vi "Dwell.vi"(8 "error in":errorcluster, 10 "Parameters":dbl[](array[numeric]), 11 "Events":i32[](array[numeric])) -> (0 "error out":errorcluster)   [LabVIEW 2013]
uses:
  NIST2/Arm Globals.vi
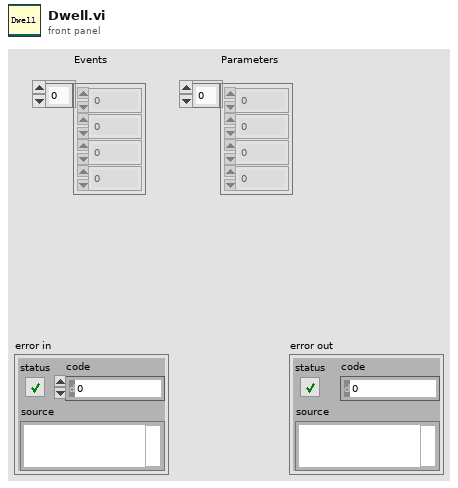
[diagram p1: front panel]
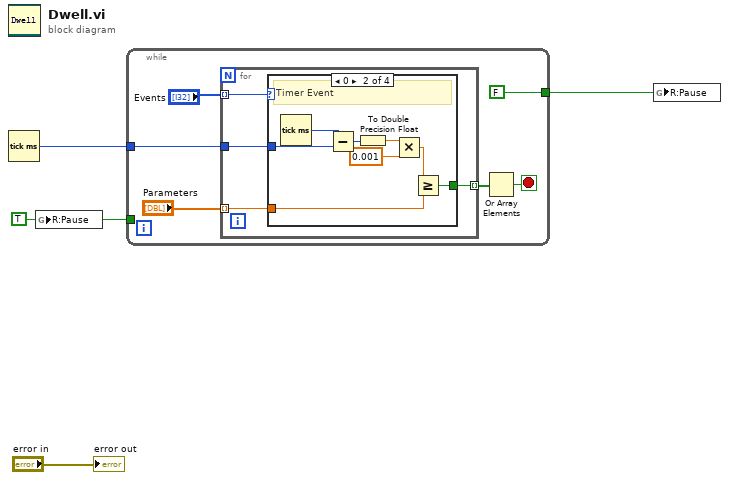
[diagram p0: block diagram]
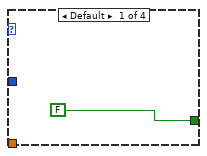
[diagram p2: hidden frame]
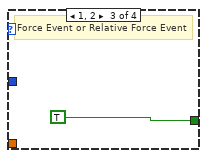
[diagram p3: hidden frame]
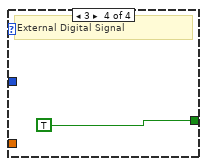
[diagram p4: hidden frame]
diagram:
  w2 = TRUE ("R:Pause")
  n1 = Tick Count (ms)() -> (millisecond timer value=w3:u32)
  n2 = global write "Arm Globals.vi" "R:Pause"(w2) -> ()
  n3 = while {
    tunnel: w3 -> [w8]
    tunnel: w2 -> [_]
    tunnel: [FALSE] -> w1
    stop <- w6 stop-if-true
    n4 = for {
      tunnel: "Events" -> [w14] mode=indexing
      tunnel: "Parameters" -> [w13] mode=indexing
      tunnel: w8 -> [w12]
      tunnel: [w11] -> w7 mode=indexing
      n5 = case shown="0" w14 {
        tunnel: w13 -> [_ w17 _ _]
        tunnel: w12 -> [_ w22 _ _]
        tunnel: [FALSE w16 TRUE TRUE] -> w11
        frame Default {
        }
        frame 0 {
          # "Timer Event"
          n6 = Tick Count (ms)() -> (millisecond timer value=w23:u32)
          n7 = Subtract(x=w23, y=w22) -> (x-y=w21:u32)
          n8 = To Double Precision Float(number=w21) -> (double precision float=w20:dbl)
          n9 = Multiply(x=w20, y=0.001) -> (x*y=w18:dbl)
          n10 = Greater Or Equal?(x=w18, y=w17) -> (x >= y?=w16:bool)
        }
        frame 1, 2 {
          # "Force Event or Relative Force Event"
        }
        frame 3 {
          # "External Digital Signal"
        }
      }
    }
    n11 = Or Array Elements(Boolean array=w7) -> (logical OR=w6:bool)
  }
  n12 = global write "Arm Globals.vi" "R:Pause"(w1) -> ()
  "error out" <- "error in"
